vi "RemoveDup.vi"(11 "Index":i32[](array[numeric])) -> (3 "DupRemoved":i32[](array[numeric]))   [LabVIEW 2014]
panel:
  out "SizeOut":i32
  out "SizeIn":i32
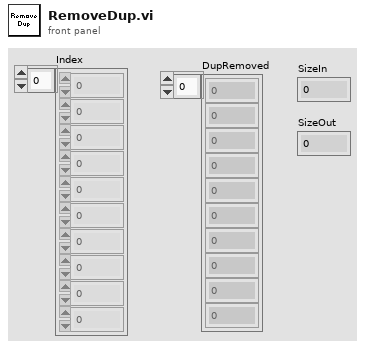
[diagram p1: front panel]
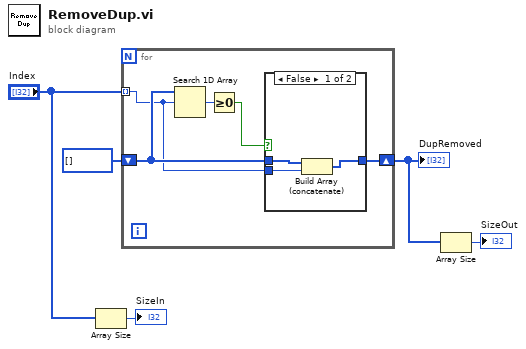
[diagram p0: block diagram]
diagram:
  n1 = Array Size(array="Index") -> (size(s)=→"SizeIn":i32)
  n2 = for {
    tunnel: "Index" -> [w6] mode=indexing
    shift-right: [w8] -> w1
    shift-left: i32[] [] -> [w7]
    n3 = Search 1D Array(1D array=w7, element=w6) -> (index of element=w10:i32)  [unwired: 1 in]
    n4 = Greater Or Equal To 0?(x=w10) -> (x >= 0?=w9:bool)
    n5 = case shown="False" w9 {
      tunnel: [w13 w14] -> w8
      tunnel: w7 -> [w12 w14]
      tunnel: w6 -> [w11 _]
      frame False {
        n6 = Build Array (concatenate)(w12, w11) -> (w13:i32[])
      }
      frame True {
      }
    }
  }
  "DupRemoved" <- w1
  n7 = Array Size(array=w1) -> (size(s)=→"SizeOut":i32)
